vi "FGV CG-Check.vi"(0 "Komponenten":u16[][](array[numeric]), 1 "Sollwerte":sgl[][](array[numeric]), 2 "Gaskonfig":T3 {"Gasflasche" items=["----"=10000, "IAG NH3 3000"=0, "IAG NH3 200"=1, "IAG NH3 2000"=2, "IAG MG"=3, "IAG O2"=4]}, 3 "max Abweichung":sgl[][](array[numeric]), 4 "Cluster":T5={"Aufschaltdauer"=0.0, "Prüfdauer"=0.0, "Mittelwertanzahl"=10} {"Prüfdauer" format="%#_5g"; "Aufschaltdauer" format="%#_5g"}, 5 "Pfad:":path=path "D:/IAG_Data/Log" caption="Path:", 6 "Analysator":T4[](array[typedef]), 7 "Aktive?":bool[](array[boolean]), 9 "Aktion":T6) -> (12 "Analysator":T4[](array[typedef]), 13 "Aktive?":bool[](array[boolean]), 14 "Komponenten":u16[][](array[numeric]), 15 "Sollwerte":sgl[][](array[numeric]), 16 "Gaskonfig":T3 {"Gasflasche" items=["----"=10000, "IAG NH3 3000"=0, "IAG NH3 200"=1, "IAG NH3 2000"=2, "IAG MG"=3, "IAG O2"=4]}, 17 "max Abweichung":sgl[][](array[numeric]), 18 "Cluster":T5, 19 "Pfad:":path)   [LabVIEW 2020, in "Erweiterte Konfig.lvlib" / "CG-Check Konfig.lvlib"]
uses:
  CG-Check Konfig.lvlib
  Aktion_CG-Check.ctl
  Visualisierungs Elemente/Auswahlfeld.ctl
  System Einstellungen V2/Gasflasche Auswahl.ctl
  System Einstellungen V2/Konfig Gasflasche.ctl
  Allgemein/allgemeine Sub-VIs.lvlib
  System Einstellungen V2/System Einstellungen V2.lvlib
panel:
  # "Mittelwertanzahl:"
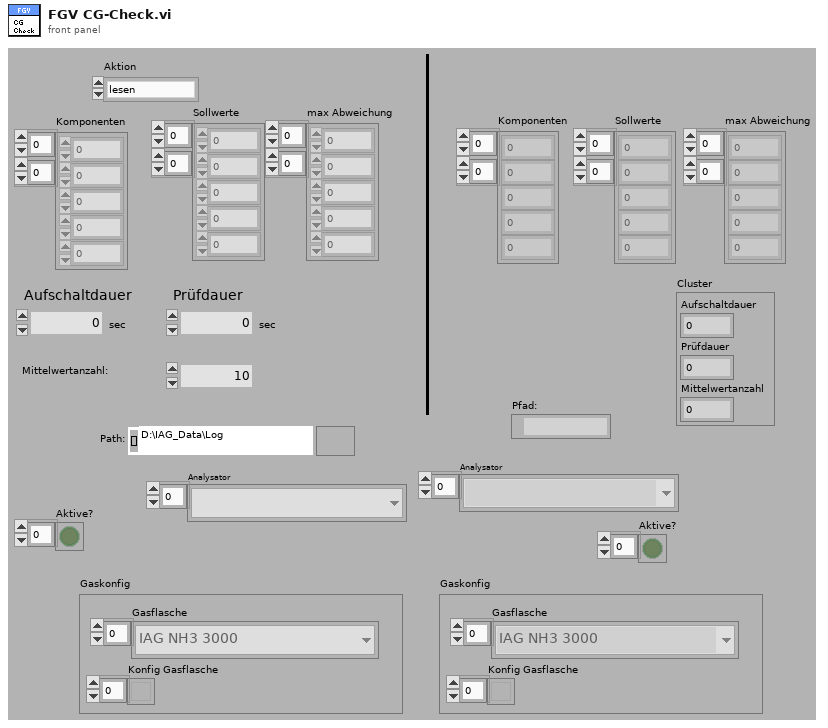
[diagram p1: front panel]
types:
  T1 = typedef "System Einstellungen V2.lvlib/Gasflasche Auswahl.ctl" = u16
  T2 = typedef "System Einstellungen V2.lvlib/Konfig Gasflasche.ctl" = bool
  T3 = cluster{"Gasflasche":T1[], "Konfig Gasflasche":T2[]}
  T4 = typedef "Auswahlfeld.ctl" = u16
  T5 = cluster{"Aufschaltdauer":sgl, "Prüfdauer":sgl, "Mittelwertanzahl":u8}
  T6 = typedef "Erweiterte Konfig.lvlib/CG-Check Konfig.lvlib/Aktion_CG-Check.ctl" = enum16{"lesen", "schreiben", "laden", "Komponente", "Aktive?", "speichern"}
  T7 = enum16{"open", "replace", "create", "open or create", "replace or create", "replace or create with confirmation"}
  T8 = cluster{"Aktive?":bool[], "Komponenten":u16[][], "Sollwerte":sgl[][], "max Abweichung":sgl[][], "Pfad:":path, "Cluster":cluster{"Aufschaltdauer":sgl, "Prüfdauer":sgl, "Mittelwertanzahl":u8}, "Analysator":T4[], "Gaskonfig":cluster{"Gasflasche":T1[], "Konfig Gasflasche":T2[]}}
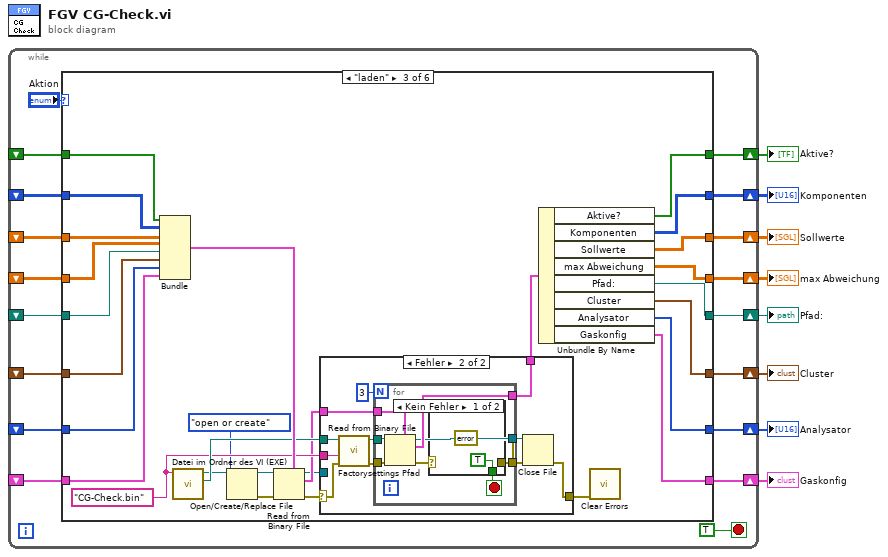
[diagram p0: block diagram]
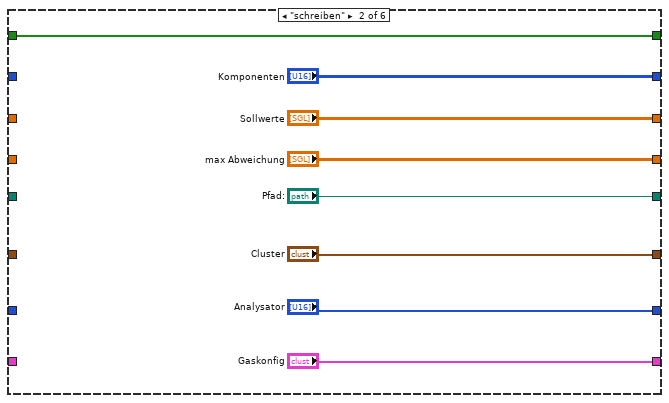
[diagram p3: hidden frame]
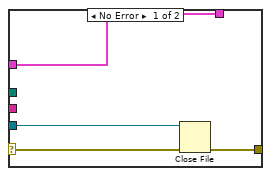
[diagram p4: hidden frame]
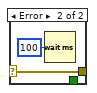
[diagram p5: hidden frame]
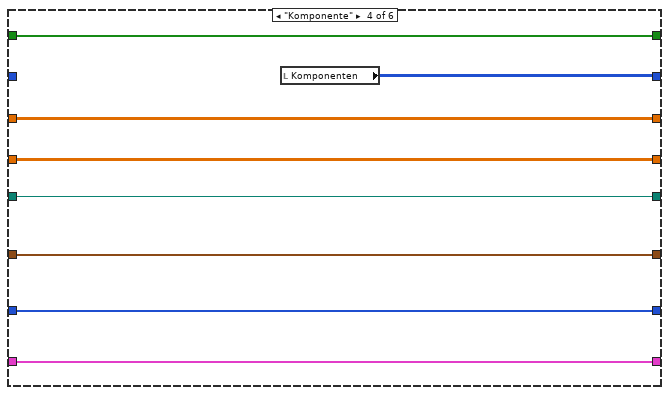
[diagram p6: hidden frame]
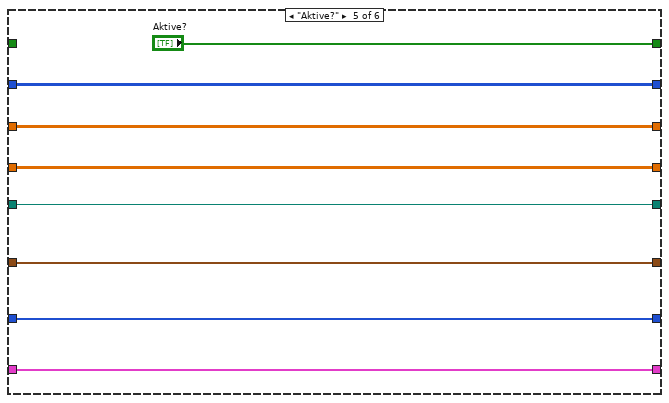
[diagram p7: hidden frame]
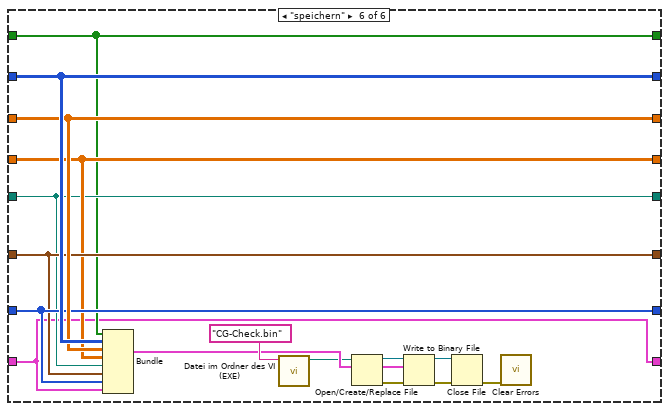
[diagram p8: hidden frame]
diagram:
  n1 = while {
    shift-right: [w24] -> w6
    shift-left: _ -> [w19]
    shift-right: [w23] -> w7
    shift-left: _ -> [w20]
    shift-right: [w22] -> w8
    shift-left: _ -> [w21]
    shift-right: [w18] -> w2
    shift-left: _ -> [w17]
    shift-right: [w15] -> w5
    shift-left: _ -> [w16]
    shift-right: [w14] -> w4
    shift-left: _ -> [w13]
    shift-right: [w12] -> w3
    shift-left: _ -> [w11]
    shift-right: [w10] -> w1
    shift-left: _ -> [w9]
    stop <- TRUE stop-if-true
    n2 = case shown="\"laden\"" "Aktion" {
      tunnel: [w32 "max Abweichung" w68 w103 w110 w123] -> w24
      tunnel: [w33 "Sollwerte" w69 w104 w111 w126] -> w23
      tunnel: [w34 "Komponenten" w70 w105 w112 w127] -> w22
      tunnel: w21 -> [w34 _ w67 _ w112 w127]
      tunnel: w20 -> [w33 _ w66 w104 w111 w126]
      tunnel: w19 -> [w32 _ w65 w103 w110 w123]
      tunnel: [w31 "Analysator" w62 w100 w107 w125] -> w18
      tunnel: w17 -> [w31 _ w63 w100 w107 w125]
      tunnel: [w30 "Cluster" w58 w101 w108 w124] -> w15
      tunnel: w16 -> [w30 _ w61 w101 w108 w124]
      tunnel: [w29 "Pfad:" w59 w102 w109 w122] -> w14
      tunnel: w13 -> [w29 _ w60 w102 w109 w122]
      tunnel: [w28 w37 w56 w99 "Aktive?" w121] -> w12
      tunnel: w11 -> [w28 w37 w57 w99 _ w121]
      tunnel: [w27 "Gaskonfig" w43 w98 w106 w114] -> w10
      tunnel: w9 -> [w27 _ w44 w98 w106 w114]
      frame "lesen", Default {
      }
      frame "schreiben" {
      }
      frame "laden" {
        w54 = "CG-Check.bin" ("Dateiname")
        n3 = Bundle("Aktive?"=w57, "Komponenten"=w67, "Sollwerte"=w66, "max Abweichung"=w65, "Pfad:"=w60, "Cluster"=w61, "Analysator"=w63, "Gaskonfig"=w44) -> (w64:T8)  [unwired: 1 in]
        n4 = call "Datei im Ordner des VI (EXE).vi"("Dateiname"=w54) -> ("Ordner des Haupt-VIs"=w55:path, "Dateipfad im Ordner des Haupt-VIs"=w47:path)  [unwired: 8 in, 1 out]
        n5 = Open/Create/Replace File(file path (use dialog)=w47, operation (0:open)=T7."open or create" ("Operation (0:open)")) -> (refnum out=w46:refnum<file>, error out=w48:errorcluster)  [unwired: 4 in, 1 out]
        n6 = Read from Binary File(5:w64, 8:w48, 11:w46) -> (0:w50:errorcluster, 2:w53:T8, 3:w49:refnum<file>)  [unwired: 4 out]
        n7 = case shown="Fehler" w50 {
          selector: w50 -> [w73 w77]
          tunnel: w55 -> [_ w78]
          tunnel: w53 -> [w74 w76]
          tunnel: [w74 w84] -> w52
          tunnel: [w71 w82] -> w51
          tunnel: w49 -> [w72 _]
          tunnel: w54 -> [_ w75]
          frame No Error {
            n8 = Close File(refnum=w72, error in=w73) -> (error out=w71:errorcluster)  [unwired: 1 out]
          }
          frame Error {
            n9 = call "Factorysettings Pfad.vi"("error in (no error)"=w77, "Dateiname"=w75, "Ordner des Haupt-VIs"=w78) -> ("error out"=w79:errorcluster, "Pfad Factorysettings"=w80:path)  [unwired: 7 in]
            n10 = for {
              N: 3 -> [_]
              tunnel: w79 -> [w91]
              tunnel: w80 -> [w90]
              tunnel: [w89] -> w84
              tunnel: [w88] -> w83
              tunnel: [w87] -> w81
              tunnel: w76 -> [w86]
              stop <- w92 stop-if-true
              n11 = Read from Binary File(5:w86, 8:w91, 11:w90) -> (0:w93:errorcluster, 2:w89:T8, 3:w87:refnum<file>)  [unwired: 3 in, 1 out]
              n12 = case shown="Kein Fehler" w93 {
                selector: w93 -> [_ w96]
                tunnel: [TRUE _] -> w92
                tunnel: [errorcluster {"status"=FALSE, "code"=0, "source"=""} ("error IO") w96] -> w88
                frame No Error {
                }
                frame Error {
                  n13 = Wait (ms)(milliseconds to wait=u32 100 ("Zu wartende ms")) -> ()  [unwired: 1 out]
                }
              }
            }
            n14 = Close File(refnum=w81, error in=w83) -> (error out=w82:errorcluster)  [unwired: 1 out]
          }
        }
        n15 = Unbundle By Name(w52) -> ("Aktive?"=w56:bool[], "Komponenten"=w70:u16[][], "Sollwerte"=w69:sgl[][], "max Abweichung"=w68:sgl[][], "Pfad:"=w59:path, "Cluster"=w58:T5, "Analysator"=w62:T4[], "Gaskonfig"=w43:T3)
        n16 = call <vilib>:"Clear Errors.vi"("error in (no error)"=w51) -> ()  [unwired: 5 in, 2 out]
      }
      frame "Komponente" {
        n17 = local read "Komponenten"() -> (w105:u16[][])
      }
      frame "Aktive?" {
      }
      frame "speichern" {
        n18 = Bundle("Aktive?"=w121, "Komponenten"=w127, "Sollwerte"=w126, "max Abweichung"=w123, "Pfad:"=w122, "Cluster"=w124, "Analysator"=w125, "Gaskonfig"=w114) -> (w128:T8)  [unwired: 1 in]
        n19 = call "Datei im Ordner des VI (EXE).vi"("Dateiname"="CG-Check.bin") -> ("Dateipfad im Ordner des Haupt-VIs"=w120:path)  [unwired: 8 in, 2 out]
        n20 = Open/Create/Replace File(file path (use dialog)=w120) -> (refnum out=w119:refnum<file>, error out=w118:errorcluster)  [unwired: 5 in, 1 out]
        n21 = Write to Binary File(file (use dialog)=w119, data=w128, error in=w118) -> (refnum out=w116:refnum<file>, error out=w117:errorcluster)  [unwired: 4 out]
        n22 = Close File(refnum=w116, error in=w117) -> (error out=w115:errorcluster)  [unwired: 1 out]
        n23 = call <vilib>:"Clear Errors.vi"("error in (no error)"=w115) -> ()  [unwired: 5 in, 2 out]
      }
    }
  }
  "Komponenten" <- w8
  "Sollwerte" <- w7
  "max Abweichung" <- w6
  "Cluster" <- w5
  "Pfad:" <- w4
  "Aktive?" <- w3
  "Analysator" <- w2
  "Gaskonfig" <- w1
